vi "Process Job.vi"(8 "error in (no error)":errorcluster, 10 "Job":refnum<class>, 11 "Mock Job Handler In":refnum<class "Mock Job Handler.lvclass">) -> (0 "error out":errorcluster, 3 "Mock Job Handler Out":refnum<class "Mock Job Handler.lvclass">)   [LabVIEW 2020, in "Mock Job Handler.lvclass"]
uses:
  Mock Job Handler.lvclass
  Mock Job Handler.lvclass/Mock Job Handler.ctl
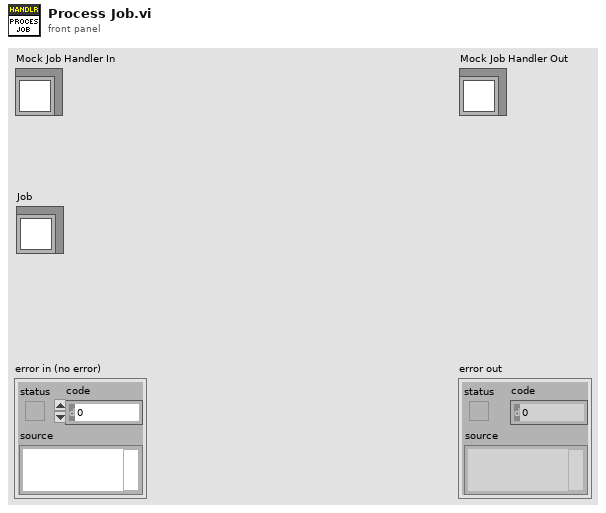
[diagram p1: front panel]
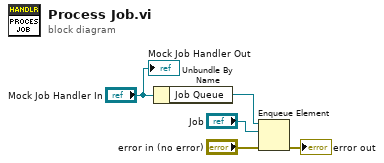
[diagram p0: block diagram]
diagram:
  n1 = Unbundle By Name("Mock Job Handler In") -> ("Job Queue"=w4:refnum<queue>)
  n2 = Enqueue Element(queue=w4, element="Job", error in (no error)="error in (no error)") -> (error out=→"error out":errorcluster)  [unwired: 1 in, 2 out]
  "Mock Job Handler Out" <- "Mock Job Handler In"
